vi "modbus__write__coil.vi"() -> ()   [LabVIEW 2020]
uses:
  <vilib>/NI/Modbus Library/API/Wrapper/Create Serial Master.vi
  <vilib>/NI/Modbus Library/API/Master/Modbus Master.lvclass
  <vilib>/NI/Modbus Library/API/Wrapper/API Main.lvlib
  <instrlib>/FlexRIO/CSI-2/API/Host/v1/NI CSI-2 API Host v1.lvlib
panel:
  in  "register to write":u16
  out "error out":errorcluster
  in  "error in":errorcluster
  in  "stop":bool
  in  "number of words":u16=1
  in  "string address":u16=1
  out "string":string
  out "data string":string
  out "string 2":string
  out "value":sgl
  in  "flow control (none)":u16(ring) items=["None", "XON/XOFF", "RTS/CTS", "XON/XOFF & RTS/CTS", "DTR/DSR", "XON/XOFF & DTR/DSR"]
  in  "parity (even)":u16(ring)=2 items=["None", "Odd", "Even", "Mark", "Space"]
  in  "serial type":enum16{"RTU", "ASCII"}(ring)
  in  "unit ID":u8=1
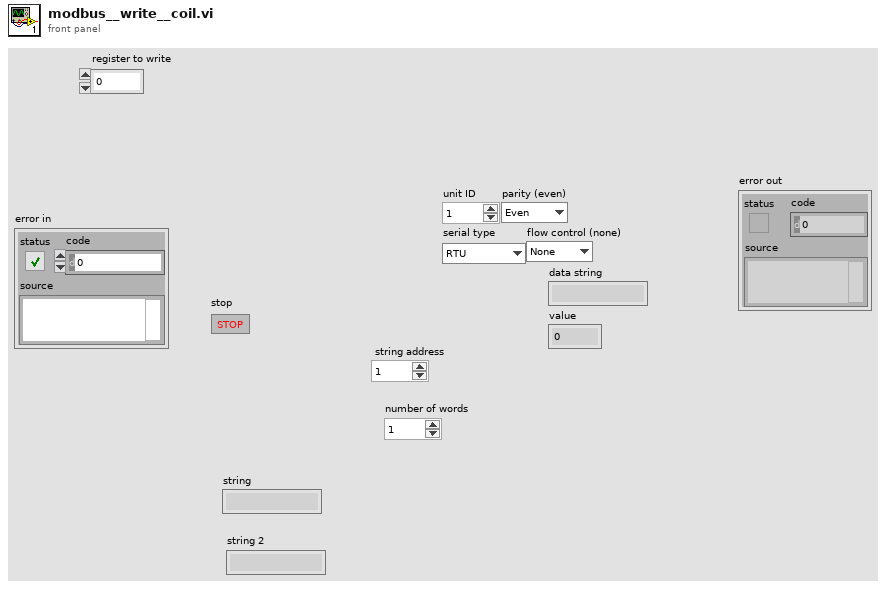
[diagram p1: front panel]
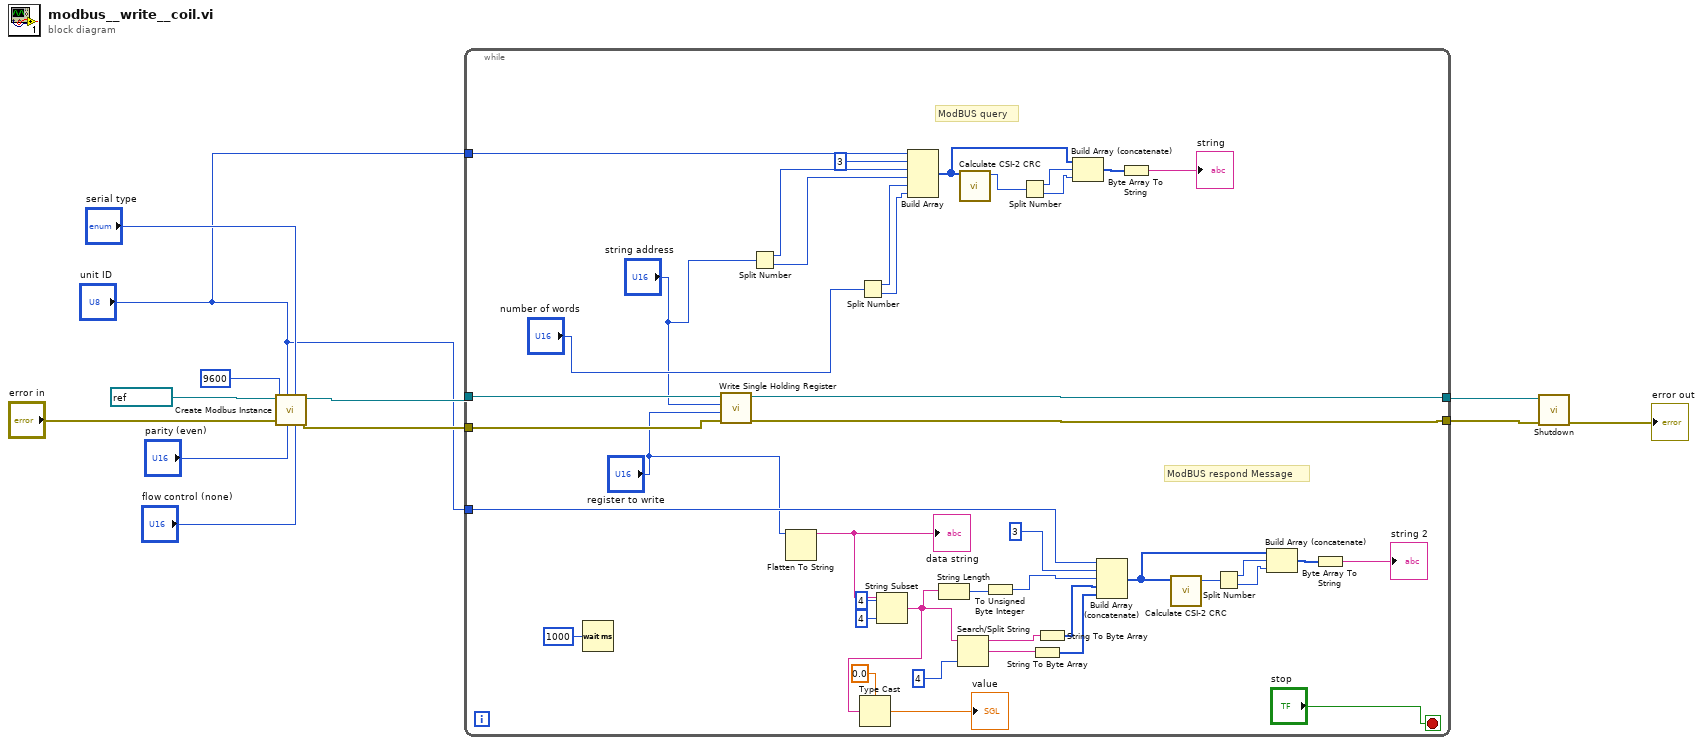
[diagram p0: block diagram]
diagram:
  n1 = call-poly <vilib>:"Create Modbus Instance.vi"("flow control (none)"="flow control (none)", "serial type"="serial type", "parity (even)"="parity (even)", "unit ID"="unit ID", "error in"="error in", "baud rate"=u32 9600, "VISA resource name"=refnum<visa-resource-name> "COM2") -> ("error out"=w7:errorcluster, "serial master instance"=w8:refnum<class "Modbus Master.lvclass">)  [unwired: 3 in]
  n2 = while {
    tunnel: [w15] -> w5
    tunnel: w8 -> [w18]
    tunnel: w7 -> [w17]
    tunnel: [w14] -> w4
    tunnel: "unit ID" -> [w53]
    tunnel: "unit ID" -> [w36]
    stop <- "stop" stop-if-true
    # "ModBUS respond Message"
    # "ModBUS query"
    n3 = Wait (ms)(milliseconds to wait=u32 1000) -> ()  [unwired: 1 out]
    n4 = call-dynamic "Write Single Holding Register.vi"("error in"=w17, "register to write"="register to write", "address"="string address", "Modbus master in"=w18) -> ("error out"=w14:errorcluster, "Modbus master out"=w15:refnum<class "Modbus Master.lvclass">)  [unwired: 6 in]
    n5 = Split Number(x="string address") -> (hi(x)=w51:u8, lo(x)=w50:u8)
    n6 = Flatten To String(anything="register to write") -> (data string=w40:string)  [unwired: 3 in, 2 out]
    "data string" <- w40
    n7 = Split Number(x="number of words") -> (hi(x)=w48:u8, lo(x)=w47:u8)
    n8 = String Subset(string=w40, offset (0)=4, length (rest)=4 ("length (rest)")) -> (substring=w23:string)
    n9 = Type Cast(type=sgl 0.0, x=w23) -> (*(type *) &x=→"value":sgl)
    n10 = Build Array(w53, u8 3 ("element"), w51, w50, w48, w47) -> (w46:u8[])
    n11 = String Length(string=w23) -> (length=w37:i32)
    n12 = Search/Split String(string=w23, offset (0)=4) -> (substring before match=w31:string, match + rest of string=w33:string)  [unwired: 1 in, 1 out]
    n13 = call <instrlib>:"Calculate CSI-2 CRC.vi"("payload"=w46) -> ("crc"=w45:u16)  [unwired: 10 in]
    n14 = To Unsigned Byte Integer(number=w37) -> (unsigned 8bit integer=w34:u8)
    n15 = Split Number(x=w45) -> (hi(x)=w44:u8, lo(x)=w43:u8)
    n16 = String To Byte Array(string=w33) -> (unsigned byte array=w29:u8[])
    n17 = String To Byte Array(string=w31) -> (unsigned byte array=w30:u8[])
    n18 = Build Array (concatenate)(w46, w44, w43) -> (w42:u8[])
    n19 = Build Array (concatenate)(w36, u8 3 ("element"), w34, w30, w29) -> (w19:u8[])
    n20 = Byte Array To String(unsigned byte array=w42) -> (string=→"string":string)
    n21 = call <instrlib>:"Calculate CSI-2 CRC.vi"("payload"=w19) -> ("crc"=w28:u16)  [unwired: 10 in]
    n22 = Split Number(x=w28) -> (hi(x)=w27:u8, lo(x)=w26:u8)
    n23 = Build Array (concatenate)(w19, w27, w26) -> (w25:u8[])
    n24 = Byte Array To String(unsigned byte array=w25) -> (string=→"string 2":string)
  }
  n25 = call-dynamic "Shutdown.vi"("error in"=w4, "Modbus master in"=w5) -> ("error out"=→"error out":errorcluster)  [unwired: 9 in]
